vi "Read Sub Panel Monedas.vi"(8 "error in (no error)":errorcluster, 11 "USD Actor in":refnum<class "USD Actor.lvclass">) -> (0 "error out":errorcluster, 2 "Sub Panel Monedas":refnum<vi>, 3 "USD Actor out":refnum<class "USD Actor.lvclass">)   [LabVIEW 2019, in "USD Actor.lvlib" / "USD Actor.lvclass"]
uses:
  USD Actor.lvclass
  USD Actor.lvclass/USD Actor.ctl
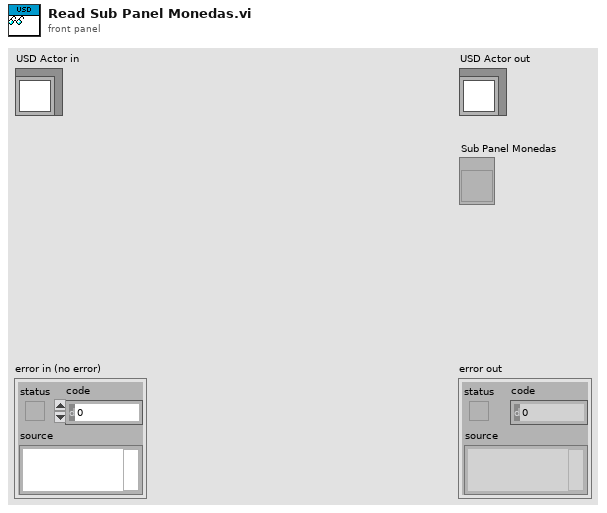
[diagram p1: front panel]
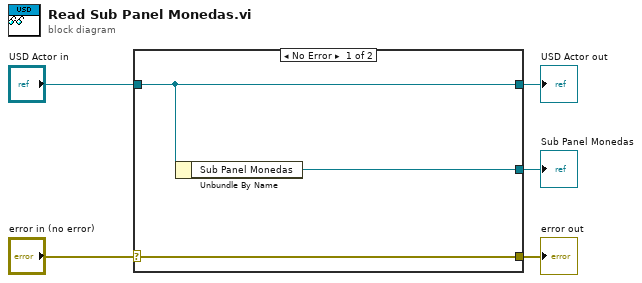
[diagram p0: block diagram]
diagram:
  n1 = case shown="No Error" "error in (no error)" {
    selector: "error in (no error)" -> [w8 w9]
    tunnel: [w8 w9] -> w4
    tunnel: [w7 w10] -> w2
    tunnel: "USD Actor in" -> [w7 w10]
    tunnel: [w6 _] -> w1
    frame No Error {
      n2 = Unbundle By Name(w7) -> ("Sub Panel Monedas"=w6:refnum<vi>)
    }
    frame Error {
    }
  }
  "error out" <- w4
  "USD Actor out" <- w2
  "Sub Panel Monedas" <- w1
